vi "Write String.vi"(10 "String":string, 11 "Caraya-TestableClass in":refnum<class "Caraya-TestableClass.lvclass">) -> (3 "Caraya-TestableClass out":refnum<class "Caraya-TestableClass.lvclass">)   [LabVIEW 2020, in "Caraya-TestableClass.lvclass"]
uses:
  Caraya-TestableClass.lvclass
  Caraya-TestableClass.lvclass/Caraya-TestableClass.ctl
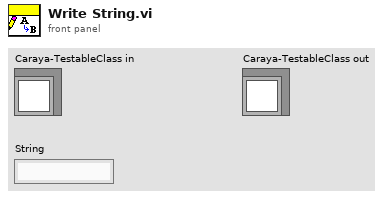
[diagram p1: front panel]
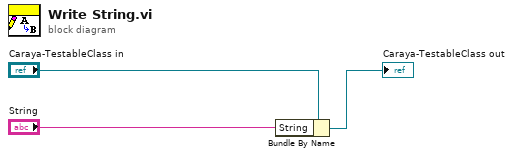
[diagram p0: block diagram]
diagram:
  n1 = Bundle By Name(cluster="Caraya-TestableClass in", "String"="String") -> (→"Caraya-TestableClass out":refnum<class "Caraya-TestableClass.lvclass">)
